vi "PH_Countdown-Counter.ProcCases.vi"(0 "i ref in":refnum<vi>, 1 "selector":string, 2 "Data":T1, 3 "call cluster":T2={"Object"="", "Selector"="", "CallType"=enum."synchronous", "Async Object"="", "Async Selector"="", "Data Descriptor"="", "Data"=[], "Error #"=0, "Expire"=0}, 5 "error in (no error)":errorcluster) -> (14 "i ref out":refnum<vi>, 17 "answer cluster":T2={"Object"="", "Selector"="", "CallType"=enum."synchronous", "Async Object"="", "Async Selector"="", "Data Descriptor"="", "Data"=[], "Error #"=0, "Expire"=0}, 19 "error out":errorcluster)   [LabVIEW 2014, in "PH_Countdown-Counter.lvlib"]
doc: "This method is called by a process from within the default case in the event loop. The methods of a class that are linked to events will be called from THIS method. Add your code here."
uses:
  PH_Countdown-Counter.lvlib
  CSCore/CSSystem/CoreDefs/CoreDefs.call_type.ctl
  CSCore/BaseProcess/BaseProcess.descriptor string definition.ctl
  CSCore/CSSystem/CoreDefs/CoreDefs.rawDataType.ctl
  CSCore/CSSystem/CoreLib/CoreLib.string 2 byte array.vi
  CSCore/BaseProcess/BaseProcess.lvlib
  CSCore/CAEObj/CAEObj.lvlib
  CSCore/CSSystem/CoreLib/CoreLib.lvlib
  PH_Common/PH_Common.lvlib
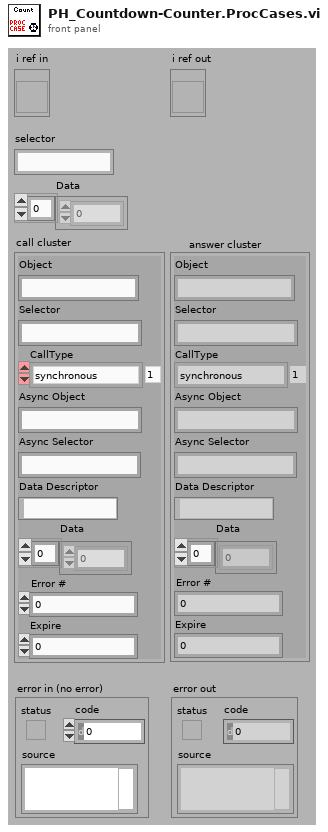
[diagram p1: front panel]
types:
  T1 = typedef "CoreDefs.rawDataType.ctl" = i8[]
  T2 = typedef "CoreDefs.call_type.ctl" = cluster{"Object":string, "Selector":string, "CallType":enum16{"simple", "synchronous", "asynchronous"}, "Async Object":string, "Async Selector":string, "Data Descriptor":T3, "Data":T1, "Error #":i32, "Expire":u32}
  T3 = typedef "BaseProcess.lvlib/BaseProcess.descriptor string definition.ctl" = string
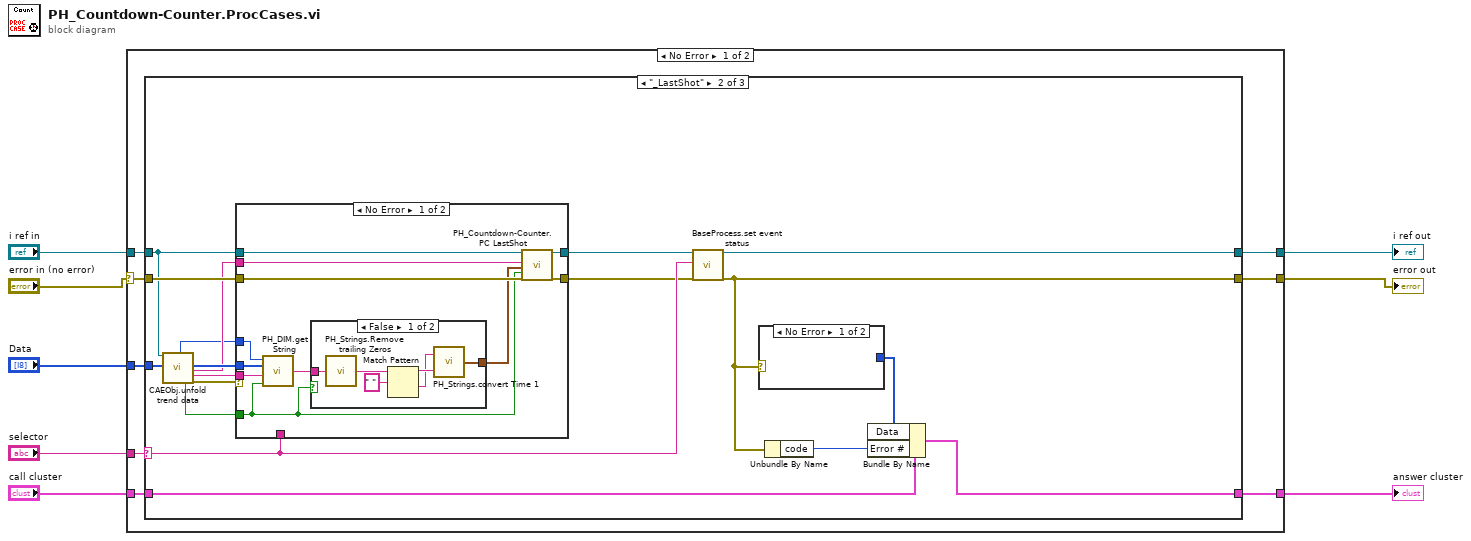
[diagram p0: block diagram]
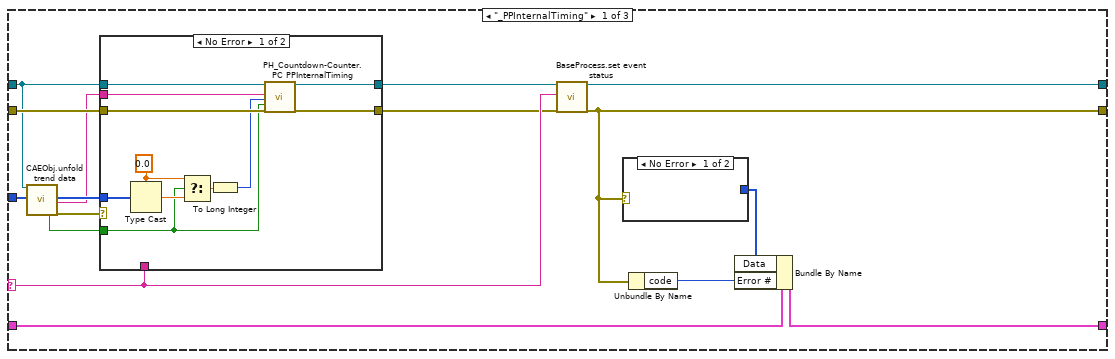
[diagram p2: hidden frame]
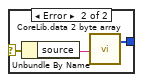
[diagram p3: hidden frame]
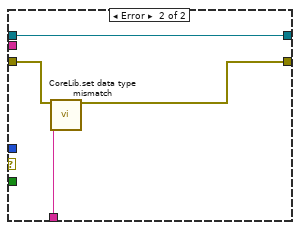
[diagram p4: hidden frame]
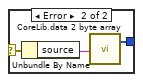
[diagram p5: hidden frame]
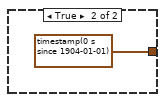
[diagram p6: hidden frame]
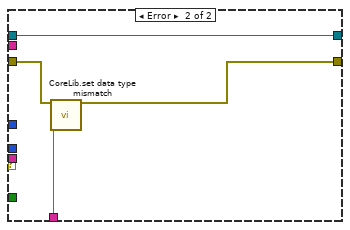
[diagram p7: hidden frame]
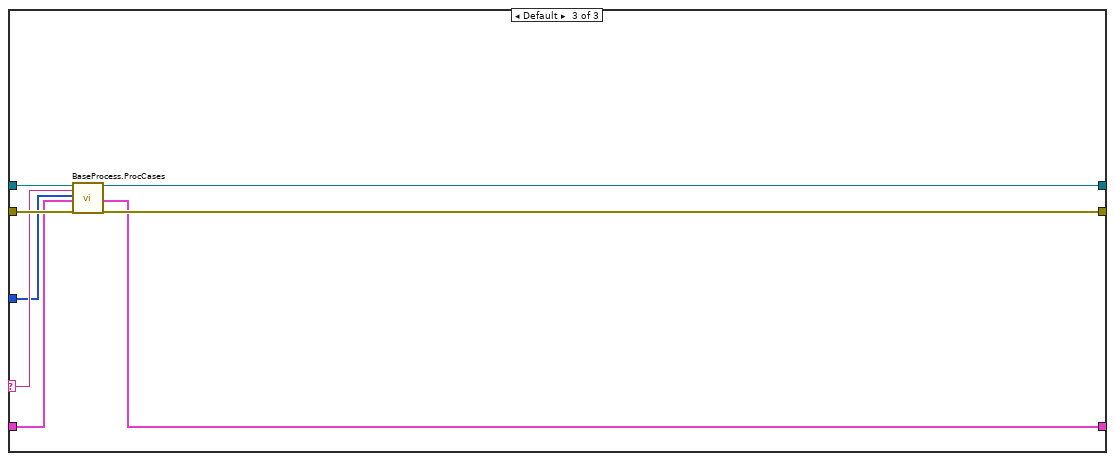
[diagram p8: hidden frame]
diagram:
  n1 = case shown="No Error" "error in (no error)" {
    selector: "error in (no error)" -> [w9 w104]
    tunnel: "selector" -> [w16 _]
    tunnel: [w15 w102] -> w7
    tunnel: "call cluster" -> [w14 w102]
    tunnel: "i ref in" -> [w13 w103]
    tunnel: [w12 w103] -> w4
    tunnel: [w11 w104] -> w3
    tunnel: "Data" -> [w10 _]
    frame No Error {
      n2 = case shown="\"_LastShot\"" w16 {
        selector: w16 -> [w29 w65 w96]
        tunnel: w13 -> [w21 w57 w95]
        tunnel: [w26 w62 w101] -> w12
        tunnel: w14 -> [w23 w59 w97]
        tunnel: [w24 w60 w98] -> w15
        tunnel: w9 -> [w32 w68 w100]
        tunnel: [w25 w61 w99] -> w11
        tunnel: w10 -> [w22 w58 w94]
        frame "_PPInternalTiming" {
          n3 = call "CAEObj.unfold trend data.vi"("i ref in"=w21, "raw trend data"=w22) -> ("no link"=w19:bool, "data"=w18:i8[], "serviceName"=w17:string, "error out"=w20:errorcluster)  [unwired: 9 in, 5 out]
          n4 = case shown="No Error" w20 {
            tunnel: [w38 w50] -> w28
            tunnel: w21 -> [w46 w50]
            tunnel: w32 -> [w45 w49]
            tunnel: [w37 w48] -> w27
            tunnel: w29 -> [_ w47]
            tunnel: w19 -> [w36 _]
            tunnel: w18 -> [w43 _]
            tunnel: w17 -> [w42 _]
            frame No Error {
              w41 = 0.0
              n5 = Type Cast(type=w41, x=w43) -> (*(type *) &x=w44:dbl)
              n6 = Select(t=w41, s=w36, f=w44) -> (s? t:f=w40:dbl)
              n7 = To Long Integer(number=w40) -> (32bit integer=w39:i32)
              n8 = call "PH_Countdown-Counter.PC PPInternalTiming.vi"("i ref in"=w46, "Servicename"=w42, "Waiting Time [s]"=w39, "no link?"=w36, "error in (no error)"=w45) -> ("i ref out"=w38:refnum<vi>, "error out"=w37:errorcluster)  [unwired: 13 in]
            }
            frame Error {
              n9 = call "CoreLib.set data type mismatch.vi"("error in (no error)"=w49, "error source"=w47) -> ("error out"=w48:errorcluster)  [unwired: 17 in]
            }
          }
          n10 = call "BaseProcess.set event status.vi"("i ref in"=w28, "EventStatus"=w29, "error in (no error)"=w27) -> ("i ref out"=w26:refnum<vi>, "error out"=w25:errorcluster)  [unwired: 14 in, 1 out]
          n11 = case shown="No Error" w25 {
            selector: w25 -> [_ w35]
            tunnel: [_ w33] -> w30
            frame No Error {
            }
            frame Error {
              n12 = Unbundle By Name(w35) -> ("source"=w34:string)
              n13 = call-poly "CoreLib.data 2 byte array.vi"("string"=w34) -> ("byteArray out"=w33:T1)  [unwired: 18 in]
            }
          }
          n14 = Unbundle By Name(w25) -> ("code"=w31:i32)
          n15 = Bundle By Name(cluster=w23, "Data"=w30, "Error #"=w31) -> (w24:T2)
        }
        frame "_LastShot" {
          n16 = call "CAEObj.unfold trend data.vi"("i ref in"=w57, "raw trend data"=w58) -> ("quality"=w51:i32, "no link"=w55:bool, "data"=w54:i8[], "serviceName"=w53:string, "typeDescriptor"=w52:string, "error out"=w56:errorcluster)  [unwired: 9 in, 3 out]
          n17 = case shown="No Error" w56 {
            tunnel: [w79 w93] -> w64
            tunnel: w57 -> [w82 w93]
            tunnel: w68 -> [w81 w92]
            tunnel: [w78 w91] -> w63
            tunnel: w65 -> [_ w90]
            tunnel: w55 -> [w73 _]
            tunnel: w54 -> [w76 _]
            tunnel: w53 -> [w80 _]
            tunnel: w52 -> [w77 _]
            tunnel: w51 -> [w75 _]
            frame No Error {
              n18 = call "PH_DIM.get String.vi"("no link"=w73, "typeDescriptor"=w77, "data"=w76, "quality"=w75) -> ("Output String"=w74:string)
              n19 = case shown="False" w73 {
                tunnel: w74 -> [w85 _]
                tunnel: [w84 timestamp(0 s since 1904-01-01) ("Time")] -> w72
                frame False {
                  n20 = call "PH_Strings.Remove trailing Zeros.vi"("Input String"=w85) -> ("Output String"=w83:string)
                  n21 = Match Pattern(string=w83, regular expression=" ") -> (before substring=w87:string, after substring=w86:string)  [unwired: 1 in, 2 out]
                  n22 = call "PH_Strings.convert Time 1.vi"("Date"=w87, "Time"=w86) -> ("Time"=w84:timestamp)
                }
                frame True {
                }
              }
              n23 = call "PH_Countdown-Counter.PC LastShot.vi"("i ref in"=w82, "Servicename"=w80, "Last Shot"=w72, "no link?"=w73, "error in (no error)"=w81) -> ("i ref out"=w79:refnum<vi>, "error out"=w78:errorcluster)  [unwired: 13 in]
            }
            frame Error {
              n24 = call "CoreLib.set data type mismatch.vi"("error in (no error)"=w92, "error source"=w90) -> ("error out"=w91:errorcluster)  [unwired: 17 in]
            }
          }
          n25 = call "BaseProcess.set event status.vi"("i ref in"=w64, "EventStatus"=w65, "error in (no error)"=w63) -> ("i ref out"=w62:refnum<vi>, "error out"=w61:errorcluster)  [unwired: 14 in, 1 out]
          n26 = case shown="No Error" w61 {
            selector: w61 -> [_ w71]
            tunnel: [_ w69] -> w66
            frame No Error {
            }
            frame Error {
              n27 = Unbundle By Name(w71) -> ("source"=w70:string)
              n28 = call-poly "CoreLib.data 2 byte array.vi"("string"=w70) -> ("byteArray out"=w69:T1)  [unwired: 18 in]
            }
          }
          n29 = Unbundle By Name(w61) -> ("code"=w67:i32)
          n30 = Bundle By Name(cluster=w59, "Data"=w66, "Error #"=w67) -> (w60:T2)
        }
        frame Default {
          # "In the default case, always call the ProcCase method of the parent class"
          n31 = call "BaseProcess.ProcCases.vi"("i ref in"=w95, "selector"=w96, "Data"=w94, "call cluster"=w97, "error in (no error)"=w100) -> ("i ref out"=w101:refnum<vi>, "answer cluster"=w98:T2, "error out"=w99:errorcluster)  [unwired: 12 in]
        }
      }
    }
    frame Error {
    }
  }
  "answer cluster" <- w7
  "i ref out" <- w4
  "error out" <- w3
